vi "UPRcontroller_v00_basedonlsmv66.vi"() -> ()   [LabVIEW 2015] (continued)
                              }
                              frame #3 {
                                # "takes all the relevant variables from the front page and puts them in a buffer structure"
                                n1289 = local read "Vy-min draw"() -> (w3985:dbl)
                                n1290 = local read "Vy-max draw"() -> (w3984:dbl)
                                n1291 = local read "Vx-min draw"() -> (w3987:dbl)
                                n1292 = local read "Vx-max draw"() -> (w3986:dbl)
                                n1293 = local read "xpixels ref"() -> (w3983:i32)
                                n1294 = local read "ypixels ref"() -> (w3982:i32)
                                n1295 = local read "ROI Type"() -> (w3981:u16)
                                n1296 = local read "srateAODOtt"() -> (w4004:dbl)
                                n1297 = local read "# of frames"() -> (w4009:i32)
                                n1298 = local read "refreshtime"() -> (w4001:dbl)
                                n1299 = local read "Pel"() -> (w3980:dbl)
                                n1300 = local read "bin"() -> (w4007:dbl)
                                n1301 = local read "Override AI buffer"() -> (w3978:bool)
                                n1302 = local read "finite samples"() -> (w4016:bool)
                                n1303 = local read "srateAODOtt"() -> (w4003:dbl)
                                n1304 = local read "srateAODOtt"() -> (w4010:dbl)
                                n1305 = local read "continuous"() -> (w4015:bool)
                                n1306 = local read "Angle ref"() -> (w3988:dbl)
                                n1307 = local read "wavdet"() -> (w4017:bool)
                                n1308 = local read "Vx-ref"() -> (w4012:dbl)
                                n1309 = local read "Vy-ref"() -> (w4014:dbl)
                                n1310 = local read "avpp"() -> (w4013:i32)
                                n1311 = call "tt_timeandsamples.vi"("bin"=w4007, "refreshtime"=w4001, "srateAODOtt"=w4004, "tot#ofsamples"=w4009) -> ("refreshrate"=w4005:dbl, "refreshbuffer"=w4006:i32, "timetracecycles"=w4011:i32)  [unwired: 5 in]
                                n1312 = local read "bin"() -> (w4008:dbl)
                                n1313 = call "2pparameters.vi"("command"="get") -> ("params out"=w4020:T12)  [unwired: 1 in]
                                n1314 = Bundle By Name(cluster=w4020, "Drawing Mode"=w3981, "measpoints"=w4009, "tt_cycles"=w4011, "refreshbuffer"=w4006, "refreshrate"=w4005, "Vx-ref"=w4012, "Vy-ref"=w4014, "srate"=w4003, "finite"=w4016, "cont"=w4015, "wavdet"=w4017, "avpp"=w4013, "srateAODO"=w4010, "bufferAI"=w4006, "bin"=w4008, "Angle Img"=w3988, "Vxminref"=w3987, "Vxmaxref"=w3986, "Vyminref"=w3985, "Vymaxref"=w3984, "Xpixels Img"=w3983, "Ypixels Img"=w3982, "Pel"=w3980, "Vz-reset"=0.0, "AIoverride"=w3978) -> (w4018:T12)
                                n1315 = Reciprocal(x=w4005) -> (1/x=w4002:dbl)
                                n1316 = local write "refreshtime"(w4002) -> ()
                                n1317 = call "2pparameters.vi"("Params in"=w4018, "command"="set") -> ()  [unwired: 1 out]
                                n1318 = local read "Voltage Clamp"() -> (w3995:bool)
                                n1319 = local read "Current Clamp"() -> (w3996:bool)
                                n1320 = local read "Vholding (mV)"() -> (w3990:sgl)
                                n1321 = local read "CC_ICgain"() -> (w3994:dbl)
                                n1322 = local read "OCgain"() -> (w3991:sgl)
                                n1323 = local read "holdon"() -> (w3989:bool)
                                n1324 = call "patchparameters.vi"("command"="get") -> ("Params out"=w3998:T16)  [unwired: 1 in]
                                n1325 = Bundle By Name(cluster=w3998, "VC"=w3995, "CC"=w3996, "CC_icg (pA/mv)"=w3994, "VC_icg (mV/mV)"=10.0, "OCG (mV/pA)"=w3991, "OVG (mV/mV)"=0.1, "Vhold (mV)"=w3990, "holdon"=w3989) -> (w3997:T16)
                                n1326 = call "patchparameters.vi"("Params in"=w3997, "command"="set") -> ()  [unwired: 1 out]
                              }
                              frame #4 {
                                # "calculating the waveform from the drawing"
                                n1327 = case shown="\"freeform contour\"" w4022 {
                                frame "Point" {
                                n1328 = call "2pparameters.vi"("command"="get") -> ("params out"=w4038:T12)  [unwired: 1 in]
                                n1329 = Unbundle By Name(w4038) -> ("Pel"=w4027:sgl, "Vx-min Img"=w4040:dbl, "VX-max Img"=w4039:dbl, "Vy-min Img"=w4042:dbl, "Vy-max Img"=w4041:dbl, "Angle Img"=w4043:dbl, "Vx-ref"=w4036:dbl, "Vy-ref"=w4035:dbl)
                                n1330 = script code="Xic=(ximax+ximin)./2;\nYic=(yimax+yimin)./2;\nx=x-Xic;\ny=y-Yic;\nxout=x.*cos(pi/180.*phi)+y.*sin(pi./180.*phi)+Xic;\nyout=-x.*sin(pi./180.*phi)+y.*cos(pi./180.*phi)+Yic;"("ximax"=w4039, "ximin"=w4040, "yimax"=w4041, "yimin"=w4042, "phi"=w4043, "x"=w4036, "y"=w4035) -> ("xout"=w4029:dbl, "yout"=w4028:dbl)  [unwired: 1 in, 1 out]
                                n1331 = call "2pparameters.vi"("command"="get") -> ("params out"=w4031:T12)  [unwired: 1 in]
                                n1332 = Bundle By Name(cluster=w4031, "P"=0.0) -> (w4034:T12)
                                n1333 = Initialize Array(w4028, w4027) -> (w4025:dbl[])
                                n1334 = Initialize Array(w4029, w4027) -> (w4024:dbl[])
                                n1335 = call "2pparameters.vi"("Params in"=w4034, "command"="set") -> ()  [unwired: 1 out]
                                n1336 = call "X-array-databuffer.vi"("array in"=w4024, "command"=enum16{"get", "set", "clear", "append"}."set") -> ()  [unwired: 2 in, 2 out]
                                n1337 = call "Y-array-databuffer.vi"("array in"=w4025, "command"=enum16{"get", "set", "clear", "append"}."set") -> ()  [unwired: 2 in, 2 out]
                                }
                                frame "Resonant Ellipse", Default {
                                n1338 = call "2pparameters.vi"("command"="get") -> ("params out"=w4058:T12)  [unwired: 1 in]
                                n1339 = Unbundle By Name(w4058) -> ("srateAODO"=w4059:sgl, "Angle Img"=w4060:dbl, "Angle draw"=w4061:dbl, "Vxmaxref"=w4062:dbl, "Vxminref"=w4063:dbl, "Xpixels Img"=w4064:i32, "Ypixels Img"=w4065:i32, "Vymaxref"=w4066:dbl, "Vyminref"=w4067:dbl, "Drawing Mode"=w4068:u16, "Pel"=w4069:sgl)
                                n1340 = Add(x=w4060, y=w4061) -> (x+y=w4044:dbl)
                                n1341 = call "ROI-databuffer.vi"("command"=enum16{"get", "set", "clear", "append"}."get") -> ("array out"=w4052:cluster{"x":sgl, "y":sgl}[])  [unwired: 4 in]
                                n1342 = call "ScanningWaveform_v4.vi"("Vy-min"=w4067, "Vy-max"=w4066, "yPixels/tPixels"=w4065, "xPixels/rPixels"=w4064, "Vx-min"=w4063, "Vx-max"=w4062, "Drawing Mode"=w4068, "Angle"=w4044, "AOrate"=w4059, "Points"=w4052, "points in ellipse"=w4069) -> ("numPixels"=w4045:dbl, "Y-WaveArray"=w4046:dbl[], "P"=w4051:dbl, "X-WaveArray"=w4047:dbl[])  [unwired: 5 in]
                                n1343 = call "Y-array-databuffer.vi"("array in"=w4046, "command"=enum16{"get", "set", "clear", "append"}."set") -> ()  [unwired: 2 in, 2 out]
                                n1344 = call "X-array-databuffer.vi"("array in"=w4047, "command"=enum16{"get", "set", "clear", "append"}."set") -> ()  [unwired: 2 in, 2 out]
                                n1345 = call "2pparameters.vi"("command"="get") -> ("params out"=w4056:T12)  [unwired: 1 in]
                                n1346 = Bundle By Name(cluster=w4056, "P"=w4051, "sAOxy"=w4045, "Pel"=w4045) -> (w4048:T12)
                                n1347 = call "2pparameters.vi"("Params in"=w4048, "command"="set") -> ()  [unwired: 1 out]
                                }
                                frame "freeform contour" {
                                n1348 = disable-structure shown="Enabled" {
                                frame Disabled {
                                # "Started writing this because old one was crashing....\nI think I found the source of the crash and was able to fix old one\n-Simon"
                                n1349 = call "2pparameters.vi"("command"="get") -> ("params out"=w4083:T12)  [unwired: 1 in]
                                n1350 = Unbundle By Name(w4083) -> ("Pel"=w4072:sgl)  [unwired: 10 out]
                                n1351 = call "ROI-databuffer.vi"("command"=enum16{"get", "set", "clear", "append"}."get") -> ("array out"=w4073:cluster{"x":sgl, "y":sgl}[])  [unwired: 4 in]
                                n1352 = call "Contour_ToVolts.vi"("N Contour Points"=w4072, "Array In"=w4073) -> ("Y Array Out"=w4070:dbl[], "X Array Out"=w4071:dbl[])  [unwired: 8 in]
                                n1353 = call "2pparameters.vi"("command"="get") -> ("params out"=w4081:T12)  [unwired: 1 in]
                                n1354 = Bundle By Name(cluster=w4081, "P"=0.0, "sAOxy"=w4072, "Pel"=w4072) -> (w4075:T12)
                                n1355 = call "Y-array-databuffer.vi"("array in"=w4070, "command"=enum16{"get", "set", "clear", "append"}."set") -> ()  [unwired: 2 in, 2 out]
                                n1356 = call "X-array-databuffer.vi"("array in"=w4071, "command"=enum16{"get", "set", "clear", "append"}."set") -> ()  [unwired: 2 in, 2 out]
                                n1357 = call "2pparameters.vi"("Params in"=w4075, "command"="set") -> ()  [unwired: 1 out]
                                }
                                frame Enabled {
                                n1358 = call "2pparameters.vi"("command"="get") -> ("params out"=w4098:T12)  [unwired: 1 in]
                                n1359 = Unbundle By Name(w4098) -> ("srateAODO"=w4099:sgl, "Angle Img"=w4100:dbl, "Angle draw"=w4101:dbl, "Vxmaxref"=w4102:dbl, "Vxminref"=w4103:dbl, "Xpixels Img"=w4104:i32, "Ypixels Img"=w4105:i32, "Vymaxref"=w4106:dbl, "Vyminref"=w4107:dbl, "Drawing Mode"=w4108:u16, "Pel"=w4109:sgl)
                                n1360 = Add(x=w4100, y=w4101) -> (x+y=w4084:dbl)
                                n1361 = call "ROI-databuffer.vi"("command"=enum16{"get", "set", "clear", "append"}."get") -> ("array out"=w4092:cluster{"x":sgl, "y":sgl}[])  [unwired: 4 in]
                                n1362 = call "ScanningWaveform_v4.vi"("Vy-min"=w4107, "Vy-max"=w4106, "yPixels/tPixels"=w4105, "xPixels/rPixels"=w4104, "Vx-min"=w4103, "Vx-max"=w4102, "Drawing Mode"=w4108, "Angle"=w4084, "AOrate"=w4099, "Points"=w4092, "points in ellipse"=w4109) -> ("numPixels"=w4085:dbl, "Y-WaveArray"=w4086:dbl[], "P"=w4091:dbl, "X-WaveArray"=w4087:dbl[])  [unwired: 5 in]
                                n1363 = call "Y-array-databuffer.vi"("array in"=w4086, "command"=enum16{"get", "set", "clear", "append"}."set") -> ()  [unwired: 2 in, 2 out]
                                n1364 = call "X-array-databuffer.vi"("array in"=w4087, "command"=enum16{"get", "set", "clear", "append"}."set") -> ()  [unwired: 2 in, 2 out]
                                n1365 = call "2pparameters.vi"("command"="get") -> ("params out"=w4096:T12)  [unwired: 1 in]
                                n1366 = Bundle By Name(cluster=w4096, "P"=w4091, "sAOxy"=w4085, "Pel"=w4085) -> (w4088:T12)
                                n1367 = call "2pparameters.vi"("Params in"=w4088, "command"="set") -> ()  [unwired: 1 out]
                                }
                                }
                                }
                                }
                              }
                              frame #5 {
                                # "set starting position"
                                n1368 = call "X-array-databuffer.vi"("command"=enum16{"get", "set", "clear", "append"}."get") -> ("array out"=w4112:dbl[])  [unwired: 3 in, 1 out]
                                n1369 = call "Y-array-databuffer.vi"("command"=enum16{"get", "set", "clear", "append"}."get") -> ("array out"=w4115:dbl[])  [unwired: 3 in, 1 out]
                                n1370 = Index Array(array=w4112, index=0) -> (element=w4111:dbl)
                                n1371 = Index Array(array=w4115, index=0) -> (element=w4110:dbl)
                                n1372 = call "setposition.vi"("Vy"=w4110, "Vx"=w4111) -> ()  [unwired: 1 in]
                              }
                              frame #6 {
                                # "rem2Ps"
                                # "A2Ps"
                                # "Al"
                                # "Rl"
                                # "Here it is writing the contour to a waveform that will be given to the AO (and also DO)"
                                n1373 = stacked-sequence {
                                seq-local: [w4136 _ _ _ _ _ _ _ _ _ _] -> [_ w4256 _ w4317 _ w4403 _ _ _ _ _]
                                seq-local: [w4137 _ _ _ _ _ _ _ _ _ _] -> [_ w4257 w4267 _ w4372 _ _ _ _ _ _]
                                seq-local: [_ _ w4266 _ _ _ _ _ _ _ _] -> [_ _ _ _ w4366 _ _ _ _ _ _]
                                seq-local: [_ _ _ w4316 _ _ _ _ _ _ _] -> [_ _ _ _ _ w4402 _ _ _ _ _]
                                seq-local: [w4133 _ _ _ _ _ _ _ _ _ _] -> [_ w4253 _ _ _ _ _ _ w4612 w4680 _]
                                seq-local: [w4132 _ _ _ _ _ _ _ _ _ _] -> [_ w4252 _ _ _ _ _ _ w4613 w4681 _]
                                seq-local: [w4139 _ _ _ _ _ _ _ _ _ _] -> [_ _ _ _ _ _ w4437 _ w4611 w4679 _]
                                seq-local: [w4135 _ _ _ _ _ _ _ _ _ _] -> [_ w4251 _ _ _ _ w4439 w4520 _ _ _]
                                seq-local: [w4134 _ _ _ _ _ _ _ _ _ _] -> [_ w4250 _ _ _ _ w4438 w4519 _ _ _]
                                seq-local: [w4138 _ _ _ _ _ _ _ _ _ _] -> [_ _ _ _ _ _ w4440 w4516 _ _ _]
                                tunnel: [_ _ w4265 _ _ _ _ _ _ _ _] -> w4130
                                tunnel: [_ _ w4264 _ _ _ _ _ _ _ _] -> w4131
                                tunnel: [w4137 _ _ _ _ _ _ _ _ _ _] -> w4129
                                tunnel: [w4136 _ _ _ _ _ _ _ _ _ _] -> w4126
                                tunnel: [_ _ _ w4315 _ _ _ _ _ _ _] -> w4127
                                tunnel: [_ _ _ w4314 _ _ _ _ _ _ _] -> w4128
                                tunnel: [w4135 _ _ _ _ _ _ _ _ _ _] -> w4121
                                tunnel: [w4134 _ _ _ _ _ _ _ _ _ _] -> w4120
                                tunnel: [_ _ _ _ _ _ w4441 _ _ _ _] -> w4119
                                tunnel: [_ _ _ _ _ _ _ w4517 _ _ _] -> w4118
                                tunnel: [w4133 _ _ _ _ _ _ _ _ _ _] -> w4122
                                tunnel: [w4132 _ _ _ _ _ _ _ _ _ _] -> w4123
                                tunnel: [_ _ _ _ _ _ _ _ w4610 _ _] -> w4124
                                tunnel: [_ _ _ _ _ _ _ _ _ w4678 _] -> w4125
                                frame #0 {
                                # "for a next version, give ome thought to\nthe possibilit of intermittently updating the\nwaveforms. it will have to be a calculation\nbased on speed of CPU and program on the one hand\nand length of measurement on the other. but then it should be possible, in principle, to \nupdate the waveform on the fly and that way cut up a longer measurement in smaller parts."
                                n1374 = stacked-sequence {
                                tunnel: [w4140 _ _ _] -> w4137
                                tunnel: [_ w4152 _ _] -> w4136
                                tunnel: [_ _ _ w4217] -> w4132
                                tunnel: [_ _ _ w4216] -> w4133
                                tunnel: [_ _ _ w4215] -> w4139
                                tunnel: [_ _ w4165 _] -> w4135
                                tunnel: [_ _ w4164 _] -> w4134
                                tunnel: [_ _ w4166 _] -> w4138
                                frame #0 {
                                n1375 = call "2pparameters.vi"("command"="get") -> ("params out"=w4146:T12)  [unwired: 1 in]
                                n1376 = call "configuration.vi"("command"="get") -> ("config out"=w4142:T14)  [unwired: 2 in, 1 out]
                                n1377 = Unbundle By Name(w4142) -> ("Voltage to Xgalvo"=w4141:i32)
                                n1378 = in-place {
                                in-place-border: w4141 -> [w4151]
                                in-place-border: [w4148] -> w4140
                                n1379 = in-place-cluster #23(w4146) -> ("aAO"=w4150:u32[])
                                n1380 = call "add channel to active arrayv2.vi"("line array in"=w4150, "line to add"=w4151) -> ("line array out"=w4149:u32[], "addition"=w4148:bool)  [unwired: 1 out]
                                n1381 = in-place-cluster #23("aAO"=w4149) -> (w4144:T12)
                                }
                                n1382 = call "2pparameters.vi"("Params in"=w4144, "command"="set") -> ()  [unwired: 1 out]
                                }
                                frame #1 {
                                n1383 = call "configuration.vi"("command"="get") -> ("config out"=w4154:T14)  [unwired: 2 in, 1 out]
                                n1384 = Unbundle By Name(w4154) -> ("Voltage to Ygalvo"=w4153:i32)
                                n1385 = call "2pparameters.vi"("command"="get") -> ("params out"=w4158:T12)  [unwired: 1 in]
                                n1386 = in-place {
                                in-place-border: w4153 -> [w4163]
                                in-place-border: [w4160] -> w4152
                                n1387 = in-place-cluster #24(w4158) -> ("aAO"=w4162:u32[])
                                n1388 = call "add channel to active arrayv2.vi"("line array in"=w4162, "line to add"=w4163) -> ("line array out"=w4161:u32[], "addition"=w4160:bool)  [unwired: 1 out]
                                n1389 = in-place-cluster #24("aAO"=w4161) -> (w4156:T12)
                                }
                                n1390 = call "2pparameters.vi"("Params in"=w4156, "command"="set") -> ()  [unwired: 1 out]
                                }
                                frame #2 {
                                n1391 = call "2pparameters.vi"("command"="get") -> ("params out"=w4169:T12)  [unwired: 1 in]
                                n1392 = Unbundle By Name(w4169) -> ("autoshutter"=w4168:bool, "wavdet"=w4167:bool)
                                n1393 = case shown="True" w4168 {
                                tunnel: [w4174 w4197] -> w4165
                                tunnel: [w4173 FALSE ("removal")] -> w4164
                                tunnel: [w4172 w4196] -> w4166
                                tunnel: w4167 -> [w4171 _]
                                frame False {
                                n1394 = case shown="False" w4171 {
                                tunnel: [FALSE ("addition") FALSE ("addition")] -> w4174
                                tunnel: [w4178 FALSE ("removal")] -> w4173
                                tunnel: [w4177 _] -> w4172
                                frame False {
                                n1395 = call "2pparameters.vi"("command"="get") -> ("params out"=w4176:T12)  [unwired: 1 in]
                                n1396 = Unbundle By Name(w4176) -> ("aAS"=w4175:u32[])
                                n1397 = in-place {
                                in-place-border: [w4183] -> w4178
                                in-place-border: [w4186] -> w4177
                                in-place-border: w4175 -> [w4185]
                                n1398 = in-place-cluster #25(w4176) -> ("aDO"=w4188:u32[])
                                n1399 = for {
                                tunnel: [w4191] -> w4184 mode=indexing
                                tunnel: [w4190] -> w4186 mode=indexing
                                shift-right: [w4192] -> w4187
                                shift-left: w4188 -> [w4193]
                                tunnel: w4185 -> [w4189] mode=indexing
                                n1400 = call "remove channel from active arrayv2.vi"("line array in"=w4193, "line to remove"=w4189) -> ("line array out"=w4192:u32[], "removal"=w4191:bool, "index"=w4190:i32)
                                }
                                n1401 = Or Array Elements(Boolean array=w4184) -> (logical OR=w4183:bool)
                                n1402 = in-place-cluster #25("aDO"=w4187) -> (w4179:T12)
                                }
                                n1403 = call "2pparameters.vi"("Params in"=w4179, "command"="set") -> ()  [unwired: 1 out]
                                }
                                frame True {
                                }
                                }
                                }
                                frame True {
                                n1404 = call "2pparameters.vi"("command"="get") -> ("params out"=w4199:T12)  [unwired: 1 in]
                                n1405 = Unbundle By Name(w4199) -> ("aAS"=w4198:u32[])
                                n1406 = in-place {
                                in-place-border: w4198 -> [w4209]
                                in-place-border: [w4205] -> w4197
                                in-place-border: [w4204] -> w4196
                                n1407 = in-place-cluster #26(w4199) -> ("aDO"=w4208:u32[])
                                n1408 = for {
                                tunnel: w4209 -> [w4214] mode=indexing
                                shift-right: [w4212] -> w4207
                                shift-left: w4208 -> [w4213]
                                tunnel: [w4211] -> w4206 mode=indexing
                                tunnel: [w4210] -> w4204 mode=indexing
                                n1409 = call "add channel to active arrayv2.vi"("line array in"=w4213, "line to add"=w4214) -> ("line array out"=w4212:u32[], "addition"=w4211:bool, "index"=w4210:i32)
                                }
                                n1410 = Or Array Elements(Boolean array=w4206) -> (logical OR=w4205:bool)
                                n1411 = in-place-cluster #26("aDO"=w4207) -> (w4201:T12)
                                }
                                n1412 = call "2pparameters.vi"("Params in"=w4201, "command"="set") -> ()  [unwired: 1 out]
                                }
                                }
                                }
                                frame #3 {
                                n1413 = local read "Measurement"() -> (w4218:T4)
                                n1414 = To Unsigned Long Integer(number=w4218) -> (unsigned 32bit integer=w4219:u32)
                                n1415 = case shown="5..7" w4219 {
                                tunnel: [FALSE ("addition") w4237] -> w4217
                                tunnel: [w4222 FALSE ("removal")] -> w4216
                                tunnel: [w4220 w4235] -> w4215
                                frame 0..4, Default {
                                n1416 = call "configuration.vi"("command"="get") -> ("config out"=w4228:T14)  [unwired: 2 in, 1 out]
                                n1417 = Unbundle By Name(w4228) -> ("LT timestamp"=w4225:u32)
                                n1418 = call "2pparameters.vi"("command"="get") -> ("params out"=w4226:T12)  [unwired: 1 in]
                                n1419 = in-place {
                                in-place-border: w4225 -> [w4234]
                                in-place-border: [w4231] -> w4222
                                in-place-border: [w4230] -> w4220
                                n1420 = in-place-cluster #27(w4226) -> ("aDO"=w4233:u32[])
                                n1421 = call "remove channel from active arrayv2.vi"("line array in"=w4233, "line to remove"=w4234) -> ("line array out"=w4232:u32[], "removal"=w4231:bool, "index"=w4230:i32)
                                n1422 = in-place-cluster #27("aDO"=w4232) -> (w4223:T12)
                                }
                                n1423 = call "2pparameters.vi"("Params in"=w4223, "command"="set") -> ()  [unwired: 1 out]
                                }
                                frame 5..7 {
                                n1424 = call "configuration.vi"("command"="get") -> ("config out"=w4243:T14)  [unwired: 2 in, 1 out]
                                n1425 = Unbundle By Name(w4243) -> ("LT timestamp"=w4240:u32)
                                n1426 = call "2pparameters.vi"("command"="get") -> ("params out"=w4241:T12)  [unwired: 1 in]
                                n1427 = in-place {
                                in-place-border: w4240 -> [w4249]
                                in-place-border: [w4246] -> w4237
                                in-place-border: [w4245] -> w4235
                                n1428 = in-place-cluster #28(w4241) -> ("aDO"=w4248:u32[])
                                n1429 = call "add channel to active arrayv2.vi"("line array in"=w4248, "line to add"=w4249) -> ("line array out"=w4247:u32[], "addition"=w4246:bool, "index"=w4245:i32)
                                n1430 = in-place-cluster #28("aDO"=w4247) -> (w4238:T12)
                                }
                                n1431 = call "2pparameters.vi"("Params in"=w4238, "command"="set") -> ()  [unwired: 1 out]
                                }
                                }
                                }
                                }
                                }
                                frame #1 {
                                n1432 = Or(x=w4256, y=w4257) -> (x .or. y?=w4255:bool)
                                n1433 = case shown="True" w4255 {
                                frame False {
                                }
                                frame True {
                                # "update GUI"
                                n1434 = call "Used AO lines.vi"() -> ("used AO names"=w4261:string[], "used AO lines"=w4263:tag[])  [unwired: 2 in]
                                n1435 = control-ref of="Analog Lines Plot"() -> (w4262:refnum<vi>)
                                n1436 = local write "Analog Used Lines"(w4263) -> ()
                                n1437 = local write "Analog Used Names"(w4261) -> ()
                                n1438 = call "prepAOWaveplot.vi"("WaveformGraph in"=w4262, "Analog Used Names"=w4261) -> ()  [unwired: 1 in]
                                }
                                }
                                n1439 = Compound Arithmetic op=OR(w4253, w4252, w4251, w4250) -> (w4254:bool)
                                n1440 = case shown="True" w4254 {
                                frame False {
                                }
                                frame True {
                                n1441 = control-ref of="Digital Lines Plot"() -> (w4258:refnum<vi>)
                                n1442 = call "Used DO lines.vi"() -> ("used DO names"=w4259:string[], "used DO lines"=w4260:tag[])  [unwired: 2 in]
                                n1443 = local write "Digital Used Lines"(w4260) -> ()
                                n1444 = local write "Digital Used Names"(w4259) -> ()
                                n1445 = call "prepDOWaveplot.vi"("DigitalGraph in"=w4258, "used DO names"=w4259) -> ()  [unwired: 1 in]
                                }
                                }
                                }
                                frame #2 {
                                n1446 = case shown="True" w4267 {
                                tunnel: [w4270 w4296] -> w4266
                                tunnel: [w4269 w4294] -> w4265
                                tunnel: [w4268 _] -> w4264
                                frame False {
                                n1447 = stacked-sequence {
                                seq-local: [w4272 _] -> [_ w4287]
                                tunnel: [w4272 _] -> w4270
                                tunnel: [w4275 _] -> w4269
                                tunnel: [w4271 _] -> w4268
                                frame #0 {
                                n1448 = call "configuration.vi"("command"="get") -> ("config out"=w4283:T14)  [unwired: 2 in, 1 out]
                                n1449 = call "waveformparamsv2.vi"("command"="get") -> ("Params out"=w4277:T17)  [unwired: 4 in, 2 out]
                                n1450 = Unbundle By Name(w4283) -> ("Voltage to Xgalvo"=w4284:i32)
                                n1451 = call "2pparameters.vi"("command"="get") -> ("params out"=w4280:T12)  [unwired: 1 in]
                                n1452 = Unbundle By Name(w4277) -> ("AO parameters"=w4276:T18)
                                n1453 = Unbundle By Name(w4280) -> ("aAO"=w4281:u32[])
                                n1454 = call "waveformsAObuffer.vi"("command"="get") -> ("AO wf out"=w4273:waveform(dbl)[])  [unwired: 1 in]
                                n1455 = Search 1D Array(1D array=w4281, element=w4284) -> (index of element=w4272:i32)  [unwired: 1 in]
                                n1456 = Index Array(array=w4273, index=w4272) -> (element=w4271:waveform(dbl))
                                n1457 = Index Array(array=w4276, index=w4272) -> (element=w4275:T19)
                                }
                                frame #1 {
                                w4288 = 0.0 ("Step size (V)")
                                n1458 = local read "Meastab"() -> (w4286:enum32{"X-Y Image", "Linescan", "Timetrace"})
                                n1459 = case shown="\"X-Y Image\", Default" w4286 {
                                tunnel: [w4290 w4291] -> w4285
                                frame "X-Y Image", Default {
                                n1460 = local read "Sampling rate"() -> (w4290:dbl)
                                }
                                frame "Timetrace" {
                                n1461 = local read "srateAODOtt"() -> (w4291:dbl)
                                }
                                }
                                n1462 = call "replace AO XYwfparam.vi"("Baseline (V)"=w4288, "Start amplitude (V)"=w4288, "Cycles"=w4288, "Repeats"=w4288, "index of AO wave"=w4287, "Step size (V)"=w4288, "DC (%)"=w4288, "Sampling frequency (Hz)"=w4285, "Period (ms)"=w4288, "Cycle length (s)"=w4288, "Pulses"=w4288, "padding value"=w4288, "Matlab wave name"=path "xwave") -> ()  [unwired: 3 in]
                                }
                                }
                                }
                                frame True {
                                w4295 = 0.0 ("Repeats")
                                n1463 = local read "Meastab"() -> (w4293:enum32{"X-Y Image", "Linescan", "Timetrace"})
                                n1464 = case shown="\"Timetrace\"" w4293 {
                                tunnel: [w4312 w4313] -> w4292
                                frame "X-Y Image", Default {
                                n1465 = local read "Sampling rate"() -> (w4312:dbl)
                                }
                                frame "Timetrace" {
                                n1466 = local read "srateAODOtt"() -> (w4313:dbl)
                                }
                                }
                                n1467 = call "2pparameters.vi"("command"="get") -> ("params out"=w4298:T12)  [unwired: 1 in]
                                n1468 = call "configuration.vi"("command"="get") -> ("config out"=w4301:T14)  [unwired: 2 in, 1 out]
                                n1469 = call "waveformparamsv2.vi"("command"="get") -> ("Params out"=w4309:T17)  [unwired: 4 in, 2 out]
                                n1470 = Unbundle By Name(w4301) -> ("Voltage to Xgalvo"=w4302:i32)
                                n1471 = Unbundle By Name(w4309) -> ("AO parameters"=w4306:T18)
                                n1472 = Unbundle By Name(w4298) -> ("aAO"=w4299:u32[])
                                n1473 = Search 1D Array(1D array=w4299, element=w4302) -> (index of element=w4296:i32)  [unwired: 1 in]
                                n1474 = Index Array(array=w4306, index=0) -> (element=w4307:T19)
                                n1475 = Bundle By Name(cluster=w4307, "AOtab"=-1.0 ("Repeats"), "Repeats"=w4295, "Cycles"=w4295, "Start amplitude (V)"=w4295, "Baseline (V)"=w4295, "Step size (V)"=w4295, "DC (%)"=w4295, "Sampling frequency (Hz)"=w4292, "Period (ms)"=w4295, "Offset (V)"=w4295, "Amplitude (V)"=w4295, "Frequency"=w4295, "Tri Repeats"=w4295, "phase shift (ms)"=w4295, "Pulses"=w4295, "Matlab wave file"=path "xwave", "padding value"=w4295) -> (w4294:T19)
                                n1476 = Build Array(w4294) -> (w4304:T18)
                                n1477 = call "waveformparamsv2.vi"("command"="add AO", "add AO"=w4304) -> ()  [unwired: 3 in, 3 out]
                                }
                                }
                                }
                                frame #3 {
                                n1478 = case shown="True" w4317 {
                                tunnel: [w4320 w4346] -> w4316
                                tunnel: [w4319 w4344] -> w4315
                                tunnel: [w4318 _] -> w4314
                                frame False {
                                n1479 = stacked-sequence {
                                seq-local: [w4322 _] -> [_ w4337]
                                tunnel: [w4322 _] -> w4320
                                tunnel: [w4325 _] -> w4319
                                tunnel: [w4321 _] -> w4318
                                frame #0 {
                                n1480 = call "configuration.vi"("command"="get") -> ("config out"=w4333:T14)  [unwired: 2 in, 1 out]
                                n1481 = call "waveformparamsv2.vi"("command"="get") -> ("Params out"=w4327:T17)  [unwired: 4 in, 2 out]
                                n1482 = Unbundle By Name(w4333) -> ("Voltage to Ygalvo"=w4334:i32)
                                n1483 = call "2pparameters.vi"("command"="get") -> ("params out"=w4330:T12)  [unwired: 1 in]
                                n1484 = Unbundle By Name(w4327) -> ("AO parameters"=w4326:T18)
                                n1485 = Unbundle By Name(w4330) -> ("aAO"=w4331:u32[])
                                n1486 = call "waveformsAObuffer.vi"("command"="get") -> ("AO wf out"=w4323:waveform(dbl)[])  [unwired: 1 in]
                                n1487 = Search 1D Array(1D array=w4331, element=w4334) -> (index of element=w4322:i32)  [unwired: 1 in]
                                n1488 = Index Array(array=w4323, index=w4322) -> (element=w4321:waveform(dbl))
                                n1489 = Index Array(array=w4326, index=w4322) -> (element=w4325:T19)
                                }
                                frame #1 {
                                w4338 = 0.0 ("Step size (V)")
                                n1490 = local read "Meastab"() -> (w4336:enum32{"X-Y Image", "Linescan", "Timetrace"})
                                n1491 = case shown="\"X-Y Image\", Default" w4336 {
                                tunnel: [w4340 w4341] -> w4335
                                frame "X-Y Image", Default {
                                n1492 = local read "Sampling rate"() -> (w4340:dbl)
                                }
                                frame "Timetrace" {
                                n1493 = local read "srateAODOtt"() -> (w4341:dbl)
                                }
                                }
                                n1494 = call "replace AO XYwfparam.vi"("Baseline (V)"=w4338, "Start amplitude (V)"=w4338, "Cycles"=w4338, "Repeats"=w4338, "index of AO wave"=w4337, "Step size (V)"=w4338, "DC (%)"=w4338, "Sampling frequency (Hz)"=w4335, "Period (ms)"=w4338, "Cycle length (s)"=w4338, "Pulses"=w4338, "padding value"=w4338, "Matlab wave name"=path "ywave") -> ()  [unwired: 3 in]
                                }
                                }
                                }
                                frame True {
                                w4345 = 0.0 ("Repeats")
                                n1495 = local read "Meastab"() -> (w4343:enum32{"X-Y Image", "Linescan", "Timetrace"})
                                n1496 = case shown="\"X-Y Image\", Default" w4343 {
                                tunnel: [w4362 w4363] -> w4342
                                frame "X-Y Image", Default {
                                n1497 = local read "Sampling rate"() -> (w4362:dbl)
                                }
                                frame "Timetrace" {
                                n1498 = local read "srateAODOtt"() -> (w4363:dbl)
                                }
                                }
                                n1499 = call "2pparameters.vi"("command"="get") -> ("params out"=w4348:T12)  [unwired: 1 in]
                                n1500 = call "configuration.vi"("command"="get") -> ("config out"=w4351:T14)  [unwired: 2 in, 1 out]
                                n1501 = call "waveformparamsv2.vi"("command"="get") -> ("Params out"=w4360:T17)  [unwired: 4 in, 2 out]
                                n1502 = Unbundle By Name(w4351) -> ("Voltage to Ygalvo"=w4352:i32)
                                n1503 = Unbundle By Name(w4360) -> ("AO parameters"=w4357:T18)
                                n1504 = Unbundle By Name(w4348) -> ("aAO"=w4349:u32[])
                                n1505 = Search 1D Array(1D array=w4349, element=w4352) -> (index of element=w4346:i32)  [unwired: 1 in]
                                n1506 = Index Array(array=w4357, index=0) -> (element=w4358:T19)
                                n1507 = Bundle By Name(cluster=w4358, "AOtab"=-1.0 ("Repeats"), "Repeats"=w4345, "Cycles"=w4345, "Start amplitude (V)"=w4345, "Baseline (V)"=w4345, "Step size (V)"=w4345, "DC (%)"=w4345, "Sampling frequency (Hz)"=w4342, "Period (ms)"=w4345, "Offset (V)"=w4345, "Amplitude (V)"=w4345, "Frequency"=w4345, "Tri Repeats"=w4345, "phase shift (ms)"=w4345, "Pulses"=w4345, "Matlab wave file"=path "ywave", "padding value"=w4345) -> (w4344:T19)
                                n1508 = Build Array(w4344) -> (w4355:T18)
                                n1509 = call "waveformparamsv2.vi"("command"="add AO", "add AO"=w4355) -> ()  [unwired: 3 in, 3 out]
                                }
                                }
                                }
                                frame #4 {
                                n1510 = call "2pparameters.vi"("command"="get") -> ("params out"=w4369:T12)  [unwired: 1 in]
                                n1511 = Unbundle By Name(w4369) -> ("wavdet"=w4368:bool, "Pel"=w4365:sgl, "refwfsize"=w4364:dbl, "srateAODO"=w4367:sgl)
                                n1512 = case shown="True" w4368 {
                                tunnel: [w4373 w4383] -> w4371
                                tunnel: w4367 -> [w4374 w4385]
                                tunnel: w4365 -> [_ w4381]
                                tunnel: w4364 -> [_ w4380]
                                frame False {
                                n1513 = call "X-array-databuffer.vi"("command"=enum16{"get", "set", "clear", "append"}."get") -> ("array out"=w4377:dbl[])  [unwired: 3 in, 1 out]
                                n1514 = Reciprocal(x=w4374) -> (1/x=w4375:sgl)
                                n1515 = Bundle By Name("Y"=w4377, "dt"=w4375) -> (w4373:waveform(dbl))  [unwired: 1 in]
                                }
                                frame True {
                                n1516 = To Double Precision Float(number=w4381) -> (double precision float=w4382:dbl)
                                n1517 = Divide(x=w4380, y=w4382) -> (x/y=w4379:dbl)
                                n1518 = Round Toward +Infinity(x=w4379) -> (ceil(x): smallest int >= x=w4378:dbl)
                                n1519 = call "X-array-databuffer.vi"("command"=enum16{"get", "set", "clear", "append"}."get") -> ("array out"=w4387:dbl[])  [unwired: 3 in, 1 out]
                                n1520 = Reciprocal(x=w4385) -> (1/x=w4386:sgl)
                                n1521 = for {
                                N: w4378 -> [_]
                                tunnel: w4387 -> [w4389]
                                tunnel: [w4389] -> w4384 mode=concatenating
                                }
                                n1522 = Bundle By Name("Y"=w4384, "dt"=w4386) -> (w4383:waveform(dbl))  [unwired: 1 in]
                                }
                                }
                                n1523 = case shown="True" w4372 {
                                tunnel: w4371 -> [w4391 w4397]
                                tunnel: w4366 -> [w4392 _]
                                frame False {
                                n1524 = call "waveformsAObuffer.vi"("command"="get") -> ("AO wf out"=w4395:waveform(dbl)[])  [unwired: 1 in]
                                n1525 = property on="refwf" class="Ring (strict)" props=["RingText", "Text"]() -> ()  [unwired: 2 in, 3 out]
                                n1526 = Replace Array Subset(array=w4395, new element=w4391, index=w4392) -> (w4390:waveform(dbl)[])
                                n1527 = call "waveformsAObuffer.vi"("AO wf in"=w4390, "command"="set") -> ()  [unwired: 1 out]
                                }
                                frame True {
                                n1528 = call "waveformsAObuffer.vi"("command"="get") -> ("AO wf out"=w4399:waveform(dbl)[])  [unwired: 1 in]
                                n1529 = Build Array (concatenate)(w4399, w4397) -> (w4396:waveform(dbl)[])
                                n1530 = call "waveformsAObuffer.vi"("AO wf in"=w4396, "command"="set") -> ()  [unwired: 1 out]
                                }
                                }
                                }
                                frame #5 {
                                n1531 = call "2pparameters.vi"("command"="get") -> ("params out"=w4411:T12)  [unwired: 1 in]
                                n1532 = Unbundle By Name(w4411) -> ("wavdet"=w4410:bool, "Pel"=w4408:sgl, "refwfsize"=w4409:dbl, "srateAODO"=w4404:sgl)
                                n1533 = To Double Precision Float(number=w4408) -> (double precision float=w4407:dbl)
                                n1534 = Divide(x=w4409, y=w4407) -> (x/y=w4406:dbl)
                                n1535 = Round Toward +Infinity(x=w4406) -> (ceil(x): smallest int >= x=w4405:dbl)
                                n1536 = case shown="False" w4410 {
                                tunnel: [w4415 w4421] -> w4401
                                tunnel: w4405 -> [_ w4418]
                                tunnel: w4404 -> [w4416 w4423]
                                frame False {
                                n1537 = call "Y-array-databuffer.vi"("command"=enum16{"get", "set", "clear", "append"}."get") -> ("array out"=w4413:dbl[])  [unwired: 3 in, 1 out]
                                n1538 = Reciprocal(x=w4416) -> (1/x=w4417:sgl)
                                n1539 = Bundle By Name("Y"=w4413, "dt"=w4417) -> (w4415:waveform(dbl))  [unwired: 1 in]
                                }
                                frame True {
                                n1540 = call "Y-array-databuffer.vi"("command"=enum16{"get", "set", "clear", "append"}."get") -> ("array out"=w4419:dbl[])  [unwired: 3 in, 1 out]
                                n1541 = Reciprocal(x=w4423) -> (1/x=w4424:sgl)
                                n1542 = for {
                                N: w4418 -> [_]
                                tunnel: w4419 -> [w4425]
                                tunnel: [w4425] -> w4422 mode=concatenating
                                }
                                n1543 = Bundle By Name("Y"=w4422, "dt"=w4424) -> (w4421:waveform(dbl))  [unwired: 1 in]
                                }
                                }
                                n1544 = case shown="False" w4403 {
                                tunnel: w4401 -> [w4428 w4433]
                                tunnel: w4402 -> [w4429 _]
                                frame False {
                                n1545 = call "waveformsAObuffer.vi"("command"="get") -> ("AO wf out"=w4431:waveform(dbl)[])  [unwired: 1 in]
                                n1546 = Replace Array Subset(array=w4431, new element=w4428, index=w4429) -> (w4426:waveform(dbl)[])
                                n1547 = call "waveformsAObuffer.vi"("AO wf in"=w4426, "command"="set") -> ()  [unwired: 1 out]
                                }
                                frame True {
                                n1548 = call "waveformsAObuffer.vi"("command"="get") -> ("AO wf out"=w4435:waveform(dbl)[])  [unwired: 1 in]
                                n1549 = Build Array (concatenate)(w4435, w4433) -> (w4432:waveform(dbl)[])
                                n1550 = call "waveformsAObuffer.vi"("AO wf in"=w4432, "command"="set") -> ()  [unwired: 1 out]
                                }
                                }
                                }
                                frame #6 {
                                n1551 = Build Array(w4439, w4438) -> (w4443:bool[])
                                n1552 = Boolean Array To Number(Boolean array=w4443) -> (number=w4442:u32)
                                n1553 = case shown="2" w4442 {
                                tunnel: w4440 -> [w4447 w4468 _ w4486]
                                tunnel: [_ w4467 _ w4484] -> w4441
                                tunnel: w4437 -> [_ _ _ _]
                                frame 1 {
                                w4457 = 0.0 ("DOtab")
                                # "This is not correctly handling the digital channel out with multichannel\nautoshutter. It should be a for loop, and add a channel with the appropriate\nname for each autoshutter channel"
                                # "remove True; add False"
                                n1554 = call "2pparameters.vi"("command"="get") -> ("params out"=w4454:T12)  [unwired: 1 in]
                                n1555 = Unbundle By Name(w4454) -> ("srateAODO"=w4450:sgl, "Pel"=w4453:sgl)
                                n1556 = call "waveformparamsv2.vi"("command"="get") -> ("Params out"=w4463:T17)  [unwired: 4 in, 2 out]
                                n1557 = Unbundle By Name(w4463) -> ("DO parameters"=w4461:T20)
                                n1558 = To Double Precision Float(number=w4450) -> (double precision float=w4448:dbl)
                                n1559 = To Double Precision Float(number=w4450) -> (double precision float=w4449:dbl)
                                n1560 = To Double Precision Float(number=w4453) -> (double precision float=w4452:dbl)
                                n1561 = Divide(x=w4449, y=w4452) -> (x/y=w4451:dbl)
                                n1562 = Index Array(array=w4461, index=0) -> (element=w4460:T21)
                                n1563 = Bundle By Name(cluster=w4460, "Digital DC (%)"=100.0, "Digital phase"=w4457, "Digital Freq (Hz)"=w4451, "Sampling frequency (Hz)"=w4448, "Digital time offset (s)"=w4457, "padding value"=0.0, "matlab wave file"=path "2Pshutter", "DOtab"=0.0) -> (w4446:T21)
                                n1564 = Array Size(array=w4447) -> (size(s)=w4445:i32)
                                n1565 = Initialize Array(w4446, w4445) -> (w4444:T20)
                                n1566 = call "waveformparamsv2.vi"("command"="add DO", "add DO"=w4444) -> ()  [unwired: 3 in, 3 out]
                                }
                                frame 2 {
                                # "remove False; add True"
                                n1567 = call "waveformparamsv2.vi"("command"="get") -> ("Params out"=w4470:T17)  [unwired: 4 in, 2 out]
                                n1568 = in-place {
                                in-place-border: w4468 -> [w4474]
                                in-place-border: [w4473] -> w4467
                                n1569 = in-place-cluster #29(w4470) -> ("DO parameters"=w4476:T20)
                                n1570 = for {
                                tunnel: w4474 -> [w4480] mode=indexing
                                tunnel: [w4477] -> w4473 mode=indexing
                                shift-right: [w4481] -> w4475
                                shift-left: w4476 -> [w4482]
                                n1571 = Delete From Array(array=w4482, length=1, index=w4480) -> (deleted portion=w4479:T20, array with subset deleted=w4481:T20)
                                n1572 = Index Array(array=w4479, index=0) -> (element=w4477:T21)
                                }
                                n1573 = in-place-cluster #29("DO parameters"=w4475) -> (w4469:T17)
                                }
                                n1574 = call "waveformparamsv2.vi"("command"="set", "Params in"=w4469) -> ()  [unwired: 3 in, 3 out]
                                }
                                frame 3, Default {
                                # "Remove True; Add True"
                                }
                                frame 0 {
                                # "remove False ; add False"
                                n1575 = call "2pparameters.vi"("command"="get") -> ("params out"=w4488:T12)  [unwired: 1 in]
                                n1576 = Unbundle By Name(w4488) -> ("autoshutter"=w4487:bool, "wavdet"=w4485:bool)
                                n1577 = case shown="True" w4487 {
                                tunnel: w4486 -> [_ w4492]
                                tunnel: w4485 -> [_ w4491]
                                tunnel: [_ w4490] -> w4484
                                frame False {
                                }
                                frame True {
                                n1578 = case shown="False" w4491 {
                                tunnel: w4492 -> [w4494 _]
                                tunnel: [w4493 _] -> w4490
                                frame False {
                                n1579 = stacked-sequence {
                                tunnel: w4494 -> [w4496 w4503]
                                tunnel: [w4495 _] -> w4493
                                frame #0 {
                                n1580 = call "waveformparamsv2.vi"("command"="get") -> ("Params out"=w4498:T17)  [unwired: 4 in, 2 out]
                                n1581 = Unbundle By Name(w4498) -> ("DO parameters"=w4497:T20)
                                n1582 = for {
                                tunnel: w4497 -> [w4502]
                                tunnel: w4496 -> [w4501] mode=indexing
                                tunnel: [w4500] -> w4495 mode=indexing
                                n1583 = Index Array(array=w4502, index=w4501) -> (element=w4500:T21)
                                }
                                }
                                frame #1 {
                                n1584 = for {
                                tunnel: w4503 -> [w4514] mode=indexing
                                w4513 = 0.0 ("padding value")
                                n1585 = call "2pparameters.vi"("command"="get") -> ("params out"=w4511:T12)  [unwired: 1 in]
                                n1586 = Unbundle By Name(w4511) -> ("srate"=w4508:sgl, "Pel"=w4510:sgl)
                                n1587 = To Double Precision Float(number=w4508) -> (double precision float=w4506:dbl)
                                n1588 = To Double Precision Float(number=w4508) -> (double precision float=w4507:dbl)
                                n1589 = To Double Precision Float(number=w4510) -> (double precision float=w4509:dbl)
                                n1590 = Divide(x=w4507, y=w4509) -> (x/y=w4505:dbl)
                                n1591 = call "replace DO wf param.vi"("Digital Freq (Hz)"=w4505, "Digital DC (%)"=100.0, "Digital phase"=w4513, "Sampling frequency (Hz)"=w4506, "Digital time offset (s)"=w4513, "index of DO wave"=w4514, "padding value"=w4513, "matlab wave file"=path "2Pshutter" ("matlab wave number")) -> ()  [unwired: 3 in]
                                }
                                }
                                }
                                }
                                frame True {
                                }
                                }
                                }
                                }
                                }
                                }
                                }
                                frame #7 {
                                n1592 = Build Array(w4520, w4519) -> (w4521:bool[])
                                n1593 = Boolean Array To Number(Boolean array=w4521) -> (number=w4518:u32)
                                n1594 = case shown="0" w4518 {
                                tunnel: w4516 -> [w4523 w4568 _ w4579]
                                tunnel: [_ w4569 _ w4577] -> w4517
                                frame 1 {
                                n1595 = call "2pparameters.vi"("command"="get") -> ("params out"=w4530:T12)  [unwired: 1 in]
                                n1596 = Unbundle By Name(w4530) -> ("wavdet"=w4531:bool, "Pel"=w4533:sgl, "refwfsize"=w4534:dbl, "srate"=w4532:sgl)
                                n1597 = call "waveformsDObuffer.vi"("command"="get") -> ("DO wf out"=w4526:digitalwaveform[])  [unwired: 1 in]
                                n1598 = case shown="False" w4531 {
                                tunnel: [w4542 w4552] -> w4528
                                tunnel: w4532 -> [w4547 w4563]
                                tunnel: w4533 -> [w4541 w4556]
                                tunnel: w4534 -> [_ w4560]
                                frame False {
                                w4545 = u16 0 items=["unsigned binary", "offset binary", "2's complement"] ("data format (offset binary)")
                                n1599 = Initialize Array(sgl 1.0, w4541) -> (w4538:sgl[])
                                n1600 = Reciprocal(x=w4547) -> (1/x=w4548:sgl)
                                n1601 = Bundle By Name("Y"=w4538, "dt"=w4548) -> (w4543:waveform(sgl))  [unwired: 1 in]
                                n1602 = call-poly <vilib>:"Analog to Digital.vi"("data format (offset binary)"=w4545, "compress digital (T)"=TRUE, "full-scale range (pk-pk)"=1.0, "resolution (16 bit)"=1, "analog waveform"=w4543) -> ("digital waveform"=w4542:digitalwaveform)  [unwired: 3 in, 3 out]
                                }
                                frame True {
                                w4555 = u16 0 items=["unsigned binary", "offset binary", "2's complement"] ("data format (offset binary)")
                                n1603 = To Double Precision Float(number=w4556) -> (double precision float=w4561:dbl)
                                n1604 = Initialize Array(sgl 1.0, w4556) -> (w4549:sgl[])
                                n1605 = Divide(x=w4560, y=w4561) -> (x/y=w4558:dbl)
                                n1606 = Round Toward +Infinity(x=w4558) -> (ceil(x): smallest int >= x=w4559:dbl)
                                n1607 = for {
                                N: w4559 -> [_]
                                tunnel: w4549 -> [w4565]
                                tunnel: [w4565] -> w4562 mode=concatenating
                                }
                                n1608 = Reciprocal(x=w4563) -> (1/x=w4564:sgl)
                                n1609 = Bundle By Name("Y"=w4562, "dt"=w4564) -> (w4553:waveform(sgl))  [unwired: 1 in]
                                n1610 = call-poly <vilib>:"Analog to Digital.vi"("data format (offset binary)"=w4555, "compress digital (T)"=TRUE, "full-scale range (pk-pk)"=1.0, "resolution (16 bit)"=1, "analog waveform"=w4553) -> ("digital waveform"=w4552:digitalwaveform)  [unwired: 3 in, 3 out]
                                }
                                }
                                n1611 = Array Size(array=w4523) -> (size(s)=w4522:i32)
                                n1612 = for {
                                N: w4522 -> [_]
                                tunnel: w4528 -> [w4537]
                                shift-right: [w4535] -> w4524
                                shift-left: w4526 -> [w4536]
                                n1613 = Build Array (concatenate)(w4536, w4537) -> (w4535:digitalwaveform[])
                                }
                                n1614 = call "waveformsDObuffer.vi"("DO wf in"=w4524, "command"="set") -> ()  [unwired: 1 out]
                                }
                                frame 2 {
                                n1615 = Sort 1D Array(array=w4568) -> (sorted array=w4567:i32[])
                                n1616 = Reverse 1D Array(array=w4567) -> (reversed array=w4566:i32[])
                                n1617 = for {
                                tunnel: w4566 -> [w4572] mode=indexing
                                tunnel: [w4571] -> w4569
                                n1618 = call "waveformsDObuffer.vi"("command"="get") -> ("DO wf out"=w4574:digitalwaveform[])  [unwired: 1 in]
                                n1619 = Delete From Array(array=w4574, length=1, index=w4572) -> (deleted portion=w4571:digitalwaveform[], array with subset deleted=w4570:digitalwaveform[])
                                n1620 = call "waveformsDObuffer.vi"("DO wf in"=w4570, "command"="set") -> ()  [unwired: 1 out]
                                }
                                }
                                frame 3, Default {
                                }
                                frame 0 {
                                n1621 = call "2pparameters.vi"("command"="get") -> ("params out"=w4581:T12)  [unwired: 1 in]
                                n1622 = Unbundle By Name(w4581) -> ("autoshutter"=w4580:bool, "wavdet"=w4578:bool)
                                n1623 = case shown="True" w4580 {
                                tunnel: w4579 -> [_ w4585]
                                tunnel: w4578 -> [_ w4584]
                                tunnel: [_ w4583] -> w4577
                                frame False {
                                }
                                frame True {
                                n1624 = case shown="False" w4584 {
                                tunnel: w4585 -> [w4588 _]
                                tunnel: [w4587 _] -> w4583
                                frame False {
                                w4595 = u16 0 items=["unsigned binary", "offset binary", "2's complement"] ("data format (offset binary)")
                                n1625 = call "2pparameters.vi"("command"="get") -> ("params out"=w4602:T12)  [unwired: 1 in]
                                n1626 = call "waveformsDObuffer.vi"("command"="get") -> ("DO wf out"=w4589:digitalwaveform[])  [unwired: 1 in]
                                n1627 = Unbundle By Name(w4602) -> ("Pel"=w4604:sgl, "srate"=w4603:sgl)
                                n1628 = Initialize Array(sgl 1.0, w4604) -> (w4590:sgl[])
                                n1629 = Reciprocal(x=w4603) -> (1/x=w4597:sgl)
                                n1630 = Bundle By Name("Y"=w4590, "dt"=w4597) -> (w4593:waveform(sgl))  [unwired: 1 in]
                                n1631 = call-poly <vilib>:"Analog to Digital.vi"("data format (offset binary)"=w4595, "compress digital (T)"=TRUE, "full-scale range (pk-pk)"=1.0, "resolution (16 bit)"=1, "analog waveform"=w4593) -> ("digital waveform"=w4600:digitalwaveform)  [unwired: 3 in, 3 out]
                                n1632 = for {
                                tunnel: w4600 -> [w4609]
                                tunnel: w4588 -> [w4606] mode=indexing
                                tunnel: [w4605] -> w4587 mode=indexing
                                shift-right: [w4607] -> w4586
                                shift-left: w4589 -> [w4608]
                                n1633 = Index Array(array=w4608, index=w4606) -> (element=w4605:digitalwaveform)
                                n1634 = Replace Array Subset(array=w4608, new element=w4609, index=w4606) -> (w4607:digitalwaveform[])
                                }
                                n1635 = call "waveformsDObuffer.vi"("DO wf in"=w4586, "command"="set") -> ()  [unwired: 1 out]
                                }
                                frame True {
                                }
                                }
                                }
                                }
                                }
                                }
                                }
                                frame #8 {
                                n1636 = Build Array(w4613, w4612) -> (w4615:bool[])
                                n1637 = Boolean Array To Number(Boolean array=w4615) -> (number=w4614:u32)
                                n1638 = case shown="0" w4614 {
                                tunnel: w4611 -> [_ w4641 _ w4653]
                                tunnel: [_ w4640 _ w4651] -> w4610
                                frame 1 {
                                w4628 = 0.0 ("DOtab")
                                n1639 = call "2pparameters.vi"("command"="get") -> ("params out"=w4626:T12)  [unwired: 1 in]
                                n1640 = call "waveformparamsv2.vi"("command"="get") -> ("Params out"=w4636:T17)  [unwired: 4 in, 2 out]
                                n1641 = Unbundle By Name(w4636) -> ("DO parameters"=w4634:T20)
                                n1642 = Unbundle By Name(w4626) -> ("srate"=w4623:sgl, "Pel"=w4625:sgl)
                                n1643 = To Double Precision Float(number=w4623) -> (double precision float=w4621:dbl)
                                n1644 = To Double Precision Float(number=w4623) -> (double precision float=w4622:dbl)
                                n1645 = To Double Precision Float(number=w4625) -> (double precision float=w4617:dbl)
                                n1646 = Divide(x=w4622, y=w4617) -> (x/y=w4624:dbl)
                                n1647 = Index Array(array=w4634, index=0) -> (element=w4633:T21)
                                n1648 = Divide(x=1.0 ("Digital DC (%)"), y=w4617) -> (x/y=w4619:dbl)
                                n1649 = Multiply(x=100.0, y=w4619) -> (x*y=w4616:dbl)
                                n1650 = Bundle By Name(cluster=w4633, "Digital DC (%)"=w4616, "Digital phase"=w4628, "Digital Freq (Hz)"=w4624, "Sampling frequency (Hz)"=w4621, "Digital time offset (s)"=w4628, "padding value"=0.0, "matlab wave file"=path "LT", "DOtab"=0.0) -> (w4631:T21)
                                n1651 = Build Array(w4631) -> (w4630:T20)
                                n1652 = call "waveformparamsv2.vi"("command"="add DO", "add DO"=w4630) -> ()  [unwired: 3 in, 3 out]
                                }
                                frame 2 {
                                n1653 = call "waveformparamsv2.vi"("command"="get") -> ("Params out"=w4643:T17)  [unwired: 4 in, 2 out]
                                n1654 = in-place {
                                in-place-border: w4641 -> [w4647]
                                in-place-border: [w4646] -> w4640
                                n1655 = in-place-cluster #30(w4643) -> ("DO parameters"=w4649:T20)
                                n1656 = Delete From Array(array=w4649, length=1, index=w4647) -> (deleted portion=w4646:T20, array with subset deleted=w4648:T20)
                                n1657 = in-place-cluster #30("DO parameters"=w4648) -> (w4642:T17)
                                }
                                n1658 = call "waveformparamsv2.vi"("command"="set", "Params in"=w4642) -> ()  [unwired: 3 in, 3 out]
                                }
                                frame 3, Default {
                                }
                                frame 0 {
                                n1659 = local read "Measurement"() -> (w4655:T4)
                                n1660 = To Unsigned Long Integer(number=w4655) -> (unsigned 32bit integer=w4654:u32)
                                n1661 = case shown="5..7" w4654 {
                                tunnel: w4653 -> [_ w4657]
                                tunnel: [_ w4656] -> w4652
                                frame 0..4, Default {
                                }
                                frame 5..7 {
                                n1662 = stacked-sequence {
                                tunnel: w4657 -> [w4659 w4668]
